vi "Pulse.vi"() -> (8 "Pulse":dbl)   [LabVIEW 2017]
doc: "This subVI has a stored array of 15,000 heart-pulse voltage measurements that were recorded every 20 milliseconds from a finger-clip sensor."
panel:
  in  "Heart Pulse":dbl[](array[numeric])=array[15000 elements] format="%.2f"
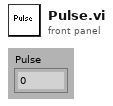
[diagram p1: front panel]
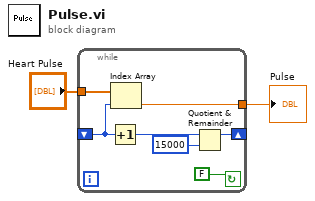
[diagram p0: block diagram]
diagram:
  n1 = while {
    shift-right: [w8] -> _
    shift-left: _ -> [w6]
    tunnel: "Heart Pulse" -> [w5]
    tunnel: [w4] -> w1
    stop <- FALSE continue-if-true
    n2 = Increment(x=w6) -> (x+1=w7:i32)
    n3 = Index Array(array=w5, index=w6) -> (element=w4:dbl)
    n4 = Quotient & Remainder(x=w7, y=15000) -> (x-y*floor(x/y)=w8:i32)  [unwired: 1 out]
  }
  "Pulse" <- w1
